vi "convertToKeyValuePair_unsignedInteger64bit.vi"(8 "error in (no error)":errorcluster, 10 "value":u64, 11 "name":string) -> (0 "error out":errorcluster, 3 "string converted":string)   [LabVIEW 2018]
doc: "Convert an 64-bit unsigned integer numeric into a key value pair as string."
uses:
  convertToKeyValuePair_string.vi
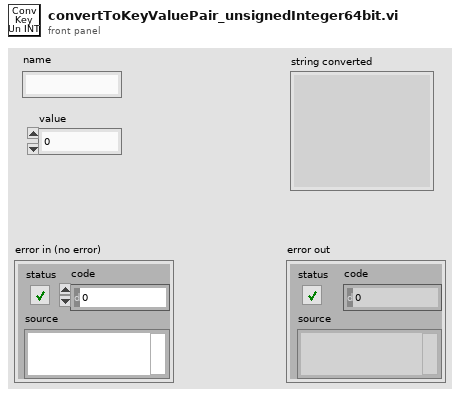
[diagram p1: front panel]
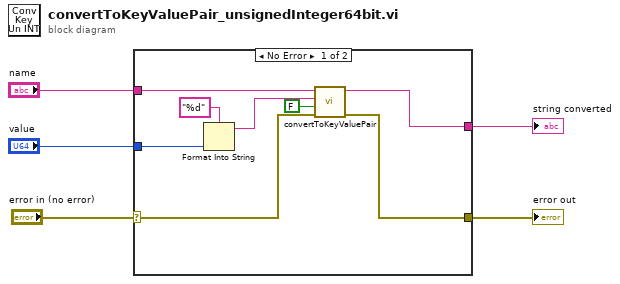
[diagram p0: block diagram]
diagram:
  n1 = case shown="No Error" "error in (no error)" {
    selector: "error in (no error)" -> [w9 w14]
    tunnel: "value" -> [w11 _]
    tunnel: "name" -> [w10 _]
    tunnel: [w8 w14] -> w2
    tunnel: [w7 _] -> w1
    frame No Error {
      n2 = Format Into String(format string="%d", w11) -> (resulting string=w13:string)  [unwired: 2 in, 1 out]
      n3 = call-poly "convertToKeyValuePair.vi"("error in (no error)"=w9, "double quotes (T)"=FALSE, "value"=w13, "name"=w10) -> ("error out"=w8:errorcluster, "string converted"=w7:string)  [unwired: 6 in]
    }
    frame Error {
    }
  }
  "error out" <- w2
  "string converted" <- w1
